vi "Read AO Data Value.vi"(8 "error in (no error)":errorcluster, 9 "Name":string, 10 "DO IOName (enum)":variant, 11 "DAQ":refnum<class "DAQ.lvclass">) -> (0 "error out":errorcluster, 2 "data value":dbl, 3 "DAQ":refnum<class "DAQ.lvclass">)   [LabVIEW 2017, in "DAQ.lvclass"]
doc: "Developed by Kevin Thompson\nkevin@thompsonengineering.net\n\nCopyright 2018-2020\nThompson Engineering, LLC"
uses:
  DAQ.lvclass
  DAQ.lvclass/DAQ.ctl
  Accessors/Get DAQ Settings.vi
  <vilib>/DAQmx/read.llb/DAQmx Read (Analog DBL 1Chan 1Samp).vi
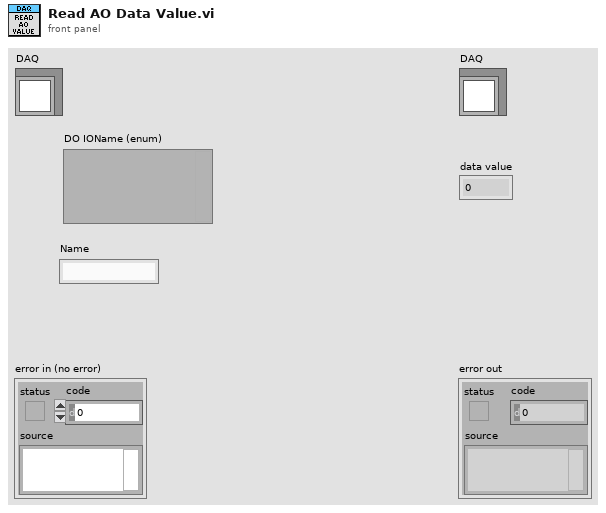
[diagram p1: front panel]
types:
  T1 = typedef "DAQ.lvclass/TD DAQ Settings--cluster.ctl" = cluster{"Simulate DAQ":bool, "DI Settings":T2[], "AI Settings":T3[], "Relay IONames":string[], "AO IONames":string[], "AO NChan SingleTask":bool}
  T2 = typedef "DAQ.lvclass/TD DI Instrument Settings--cluster.ctl" = cluster{"Disable":bool, "DI TaskName":string, "DI RefreshIntv":i32}
  T3 = typedef "DAQ.lvclass/TD AI Instrument Settings--cluster.ctl" = cluster{"Disable":bool, "AI TaskName":string, "AI InstSettings":T4, "SimAI Ranges":T5}
  T4 = typedef "DAQ.lvclass/TD AI InstSettings--cluster.ctl" = cluster{"DaqRate":dbl, "NumSamples":i32}
  T5 = typedef "DAQ.lvclass/TD SimAI Ranges--cluster.ctl" = cluster{"lo":dbl, "hi":dbl}
  T6 = typedef "DAQ.lvclass/TD AO Channel--cluster.ctl" = cluster{"DevName":string, "IOName":string, "IOPath":string, "SchemName":string, "Vmin":dbl, "Vmax":dbl, "Conversion":T7, "DAQmx Task":refnum<k21>}
  T7 = typedef "DAQ.lvclass/TD DataValueConversion--cluster.ctl" = cluster{"MaxSignal":dbl, "MinSignal":dbl, "MaxEngUnit":dbl, "MinEngUnit":dbl, "ScaleOffset":dbl, "negate":bool}
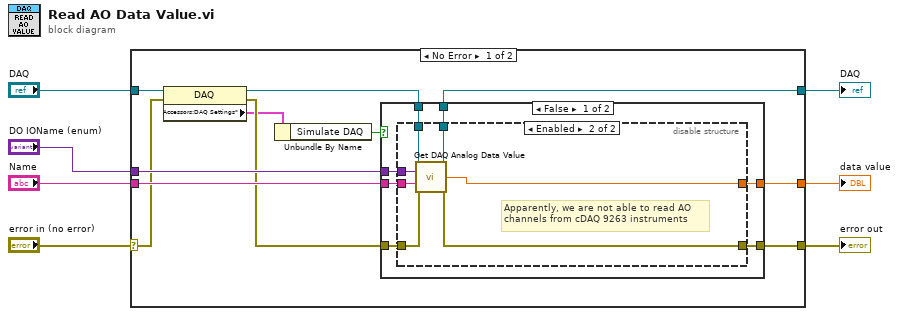
[diagram p0: block diagram]
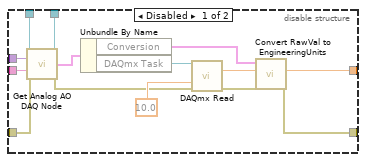
[diagram p2: hidden frame]
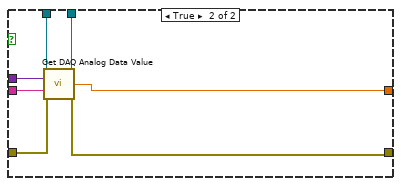
[diagram p3: hidden frame]
diagram:
  n1 = case shown="No Error" "error in (no error)" {
    selector: "error in (no error)" -> [w11 w55]
    tunnel: [w14 w55] -> w6
    tunnel: [w18 w54] -> w4
    tunnel: "DAQ" -> [w12 w54]
    tunnel: "Name" -> [w17 _]
    tunnel: "DO IOName (enum)" -> [w16 _]
    tunnel: [w15 _] -> w1
    frame No Error {
      n2 = property class="DAQ"(reference=w12, error in=w11) -> (reference out=w8:refnum<class "DAQ.lvclass">, error out=w10:errorcluster, "Accessors:DAQ Settings*"=w9:T1)
      n3 = Unbundle By Name(w9) -> ("Simulate DAQ"=w13:bool)
      n4 = case shown="False" w13 {
        tunnel: [w25 w49] -> w18
        tunnel: w17 -> [w24 w52]
        tunnel: w16 -> [w23 w53]
        tunnel: w10 -> [w22 w51]
        tunnel: [w21 w47] -> w15
        tunnel: [w20 w48] -> w14
        tunnel: w8 -> [w19 w50]
        frame False {
          n5 = disable-structure shown="Enabled" {
            disable-tunnel: [w39 w43] -> w25
            disable-tunnel: w24 -> [w38 w46]
            disable-tunnel: w23 -> [w37 w45]
            disable-tunnel: w22 -> [w36 w42]
            disable-tunnel: [w30 w40] -> w21
            disable-tunnel: [w29 w41] -> w20
            disable-tunnel: w19 -> [w26 w44]
            frame Disabled {
              n6 = call "Get Analog AO DAQ Node.vi"("DAQ"=w26, "IOName (enum)"=w37, "Name"=w38, "error in (no error)"=w36) -> ("DAQ"=w39:refnum<class "DAQ.lvclass">, "AO DAQNode out"=w35:T6, "error out"=w32:errorcluster)  [unwired: 9 in]
              n7 = Unbundle By Name(w35) -> ("Conversion"=w27:T7, "DAQmx Task"=w34:refnum<k21>)
              n8 = call-poly <vilib>:"DAQmx Read.vi"("task/channels in"=w34, "timeout"=10.0, "error in"=w32) -> ("data"=w31:dbl, "error out"=w28:errorcluster)  [unwired: 10 in, 1 out]
              n9 = call "Convert RawVal to EngineeringUnits.vi"("error in (no error)"=w28, "Raw Value In"=w31, "Conversion"=w27) -> ("error out"=w29:errorcluster, "Engineering Units Out"=w30:dbl)  [unwired: 7 in]
            }
            frame Enabled {
              # "Apparently, we are not able to read AO\nchannels from cDAQ 9263 instruments"
              n10 = call "Get DAQ Analog Data Value.vi"("DAQ"=w44, "IOName (enum)"=w45, "Name"=w46, "error in (no error)"=w42) -> ("DAQ"=w43:refnum<class "DAQ.lvclass">, "Value"=w40:dbl, "error out"=w41:errorcluster)  [unwired: 9 in]
            }
          }
        }
        frame True {
          n11 = call "Get DAQ Analog Data Value.vi"("DAQ"=w50, "IOName (enum)"=w53, "Name"=w52, "error in (no error)"=w51) -> ("DAQ"=w49:refnum<class "DAQ.lvclass">, "Value"=w47:dbl, "error out"=w48:errorcluster)  [unwired: 9 in]
        }
      }
    }
    frame Error {
    }
  }
  "error out" <- w6
  "DAQ" <- w4
  "data value" <- w1
